vi "GetDisplayName.vi"(8 "error in (no error)":errorcluster, 11 "CDefaultRuleFileParser in":refnum<class "CDefaultRuleFileParser.lvclass">) -> (0 "error out":errorcluster, 1 "Display name":string, 3 "CDefaultRuleFileParser out":refnum<class "CDefaultRuleFileParser.lvclass">)   [LabVIEW 2020, in "DefaultExtensions.lvlib" / "CDefaultRuleFileParser.lvclass"]
uses:
  CDefaultRuleFileParser.lvclass
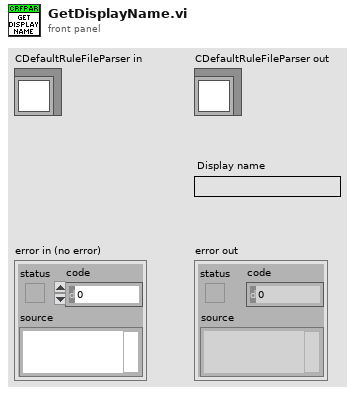
[diagram p1: front panel]
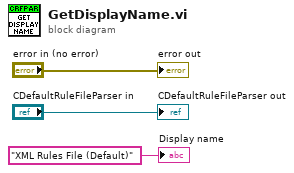
[diagram p0: block diagram]
diagram:
  "error out" <- "error in (no error)"
  "CDefaultRuleFileParser out" <- "CDefaultRuleFileParser in"
  "Display name" <- "XML Rules File (Default)" ("Display name")
